vi "Create Timing Channel Array.vi"(11 "timing channel ref":T1 format="%.0x") -> (2 "channel offset":i64, 3 "timing channel ref array":T1[](array[typedef]) format="%.0x")   [LabVIEW 2024, in "AIM ARINC 429 Engine.lvlib" / "Implementation.lvlib" / "Execution Unit Factory.lvclass"]
uses:
  Execution Unit Factory.lvclass
  <vilib>/NI VeriStand/Custom Device API/Custom Device Item Ref.ctl
  <vilib>/NI VeriStand/Custom Device API/Custom Device API.lvlib
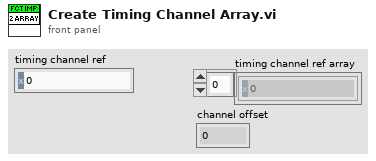
[diagram p1: front panel]
types:
  T1 = typedef "Custom Device API.lvlib/Custom Device Item Ref.ctl" = u64
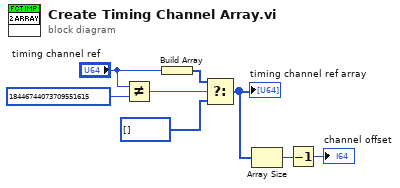
[diagram p0: block diagram]
diagram:
  n1 = Not Equal?(x="timing channel ref", y=T1 18446744073709551615) -> (x != y?=w7:bool)
  n2 = Build Array("timing channel ref") -> (w5:T1[])
  n3 = Select(t=w5, s=w7, f=T1[] []) -> (s? t:f=w3:T1[])
  "timing channel ref array" <- w3
  n4 = Array Size(array=w3) -> (size(s)=w2:i32)
  n5 = Decrement(x=w2) -> (x-1=→"channel offset":i32)
